vi "Pop Content.vi"(8 "Error In":errorcluster, 10 "Characters Count":i32=1, 11 "Parser In":refnum<class "Parser.lvclass">) -> (0 "Error Out":errorcluster, 3 "Parser Out":refnum<class "Parser.lvclass">)   [LabVIEW 2018, in "Toolkit.lvlib" / "Parser.lvclass"]
uses:
  Parser.lvclass
  Parser.lvclass/Parser.ctl
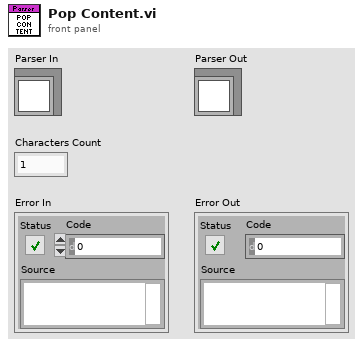
[diagram p1: front panel]
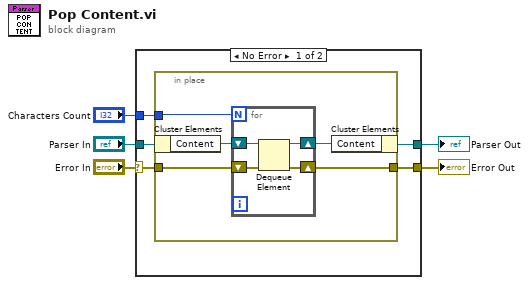
[diagram p0: block diagram]
diagram:
  n1 = case shown="No Error" "Error In" {
    selector: "Error In" -> [w6 w20]
    tunnel: [w10 w20] -> w5
    tunnel: "Characters Count" -> [w9 _]
    tunnel: [w8 w21] -> w3
    tunnel: "Parser In" -> [w7 w21]
    frame No Error {
      n2 = in-place {
        in-place-border: w6 -> [w14]
        in-place-border: w9 -> [w13]
        in-place-border: [w11] -> w10
        n3 = in-place-cluster #1(w7) -> ("Content"=w15:refnum<queue>)
        n4 = for {
          N: w13 -> [_]
          shift-right: [w18] -> w12
          shift-left: w15 -> [w19]
          shift-right: [w16] -> w11
          shift-left: w14 -> [w17]
          n5 = Dequeue Element(queue=w19, error in (no error)=w17) -> (queue out=w18:refnum<queue>, error out=w16:errorcluster)  [unwired: 1 in, 2 out]
        }
        n6 = in-place-cluster #1("Content"=w12) -> (w8:refnum<class "Parser.lvclass">)
      }
    }
    frame Error {
    }
  }
  "Error Out" <- w5
  "Parser Out" <- w3
